vi "Gif.ExtractTime.vi"(2 "GraphicControlExtension":T1, 9 "offset":i32, 11 "error in (no error)":errorcluster) -> (4 "time":u32, 10 "offset out":i32, 15 "error out":errorcluster)   [LabVIEW 2019]
uses:
  Gif.GraphicControlExtension.ctl
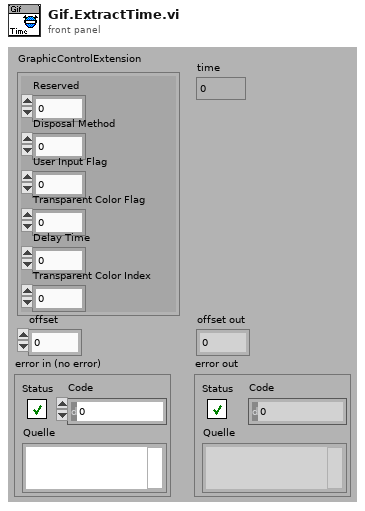
[diagram p1: front panel]
types:
  T1 = typedef "Gif.GraphicControlExtension.ctl" = cluster{"Reserved":u8, "Disposal Method":u8, "User Input Flag":u8, "Transparent Color Flag":u8, "Delay Time":u16, "Transparent Color Index":u8}
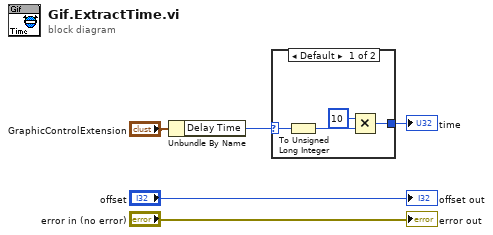
[diagram p0: block diagram]
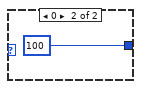
[diagram p2: hidden frame]
diagram:
  n1 = Unbundle By Name("GraphicControlExtension") -> ("Delay Time"=w3:u16)
  n2 = case shown="Default" w3 {
    selector: w3 -> [w8 _]
    tunnel: [w9 u32 100] -> w5
    frame Default {
      n3 = To Unsigned Long Integer(number=w8) -> (unsigned 32bit integer=w6:u32)
      n4 = Multiply(x=u32 10 ("t"), y=w6) -> (x*y=w9:u32)
    }
    frame 0 {
    }
  }
  "time" <- w5
  "error out" <- "error in (no error)"
  "offset out" <- "offset"
